vi "Vision Processing.vi"(4 "error in (no error)":errorcluster, 7 "Image Size":T1=enum."320x240") -> ()   [LabVIEW 2013]
doc: "This VI runs in parallel to other tasks. It gets images from the camera, processes them for color or shape and use that information to affect robot behavior."
uses:
  <vilib>/Rock Robotics/WPI/Camera/WPI_CameraImageSize.ctl
  <vilib>/Rock Robotics/WPI/Camera/WPI_CameraWhite Balance Values.ctl
  <vilib>/Rock Robotics/WPI/Camera/WPI_CameraExposure Values.ctl
  <vilib>/Rock Robotics/WPI/Camera/WPI_CameraFrameRate.ctl
  Robot Global Data.vi
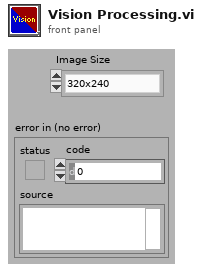
[diagram p1: front panel]
types:
  T1 = typedef "WPI_CameraImageSize.ctl" = enum16{"640x480", "320x240", "160x120"}
  T2 = typedef "WPI_CameraFrameRate.ctl" = u32
  T3 = typedef "WPI_CameraExposure Values.ctl" = enum16{"Auto", "Flicker-free 50 Hz", "Flicker-free 60 Hz", "Hold current"}
  T4 = typedef "WPI_CameraWhite Balance Values.ctl" = enum16{"Auto", "Fixed indoor", "Fixed outdoor 1", "Fixed outdoor 2", "Fixed fluorescent 1", "Fixed fluorescent 2", "Hold current"}
  T5 = typedef "Image Type" = u32
  T6 = typedef "WPI_CameraDevRef.ctl" = cluster{"Camera Address":string, "CameraStatus":errorcluster, "Acquire Image Notifier":refnum<notifier>}
  T7 = typedef "IMAQ Image.ctl" = refnum<image>
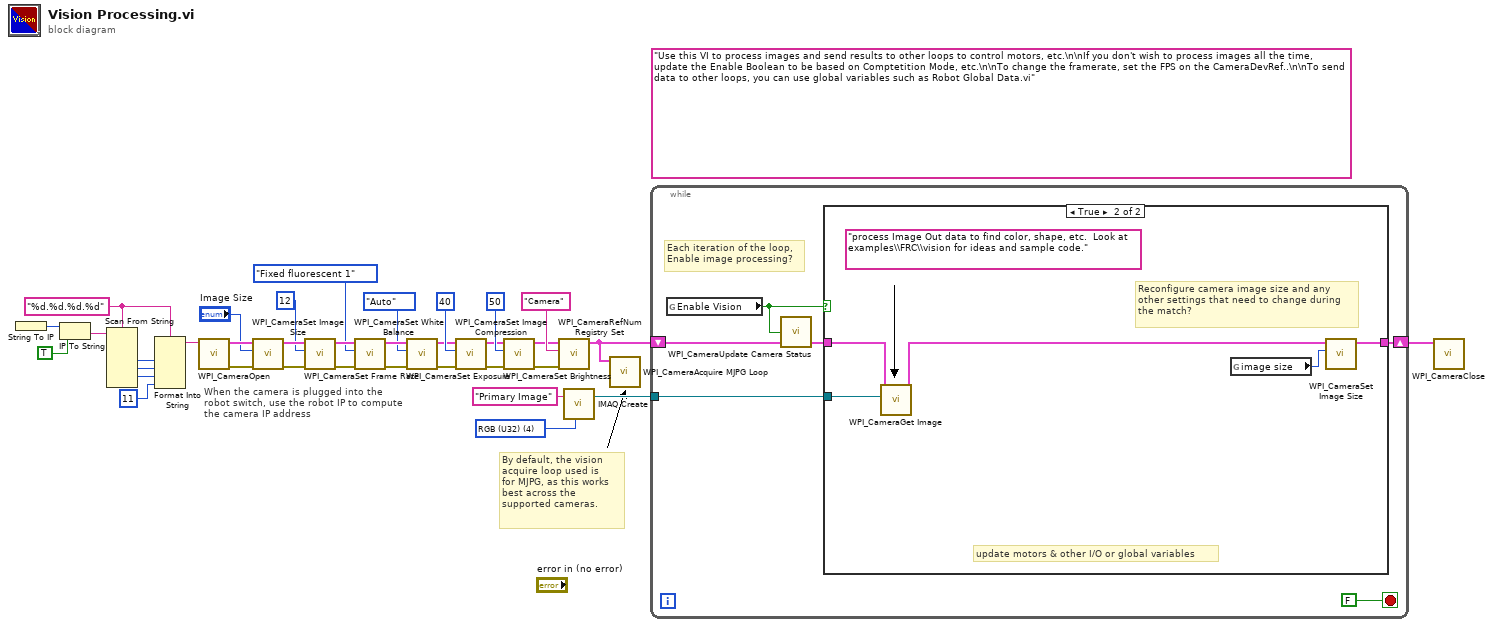
[diagram p0: block diagram]
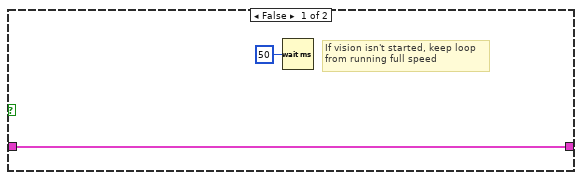
[diagram p2: hidden frame]
diagram:
  w5 = "%d.%d.%d.%d" ("format string")
  (unwired) "Use this VI to process images and send results to other loops to control motors, etc.\n\nIf you don't wish to process images all the time, update the Enable Boolean to be based on Comptetition Mode, etc.\n\nTo change the framerate, set the FPS on the CameraDevRef..\n\nTo send data to other loops, you can use global variables such as Robot Global Data.vi"
  w35 = T5 4 items=["Grayscale (U8)", "Grayscale (I16)", "Grayscale (SGL)", "Complex (CSG)", "RGB (U32)", "HSL (U32)", "RGB (U64)"] ("Image Type")
  # "When the camera is plugged into the\nrobot switch, use the robot IP to compute\nthe camera IP address"
  # "By default, the vision\nacquire loop used is\nfor MJPG, as this works\nbest across the\nsupported cameras."
  n1 = String To IP() -> (0:w12:u32)  [unwired: 1 in]
  n2 = IP To String(1:TRUE ("dot notation? (F)"), 2:w12) -> (0:w10:string)
  n3 = Scan From String(format string=w5, input string=w10) -> (output 1=w9:i32, output 2=w8:i32, output 3=w7:i32)  [unwired: 7 in, 3 out]
  n4 = Format Into String(format string=w5, w9, w8, w7, 11 ("Compression")) -> (resulting string=w4:string)  [unwired: 2 in, 1 out]
  n5 = call <vilib>:"WPI_CameraOpen.vi"("Camera Address"=w4) -> ("error out"=w23:errorcluster, "CameraDevRef"=w24:T6)  [unwired: 1 in, 8 out]
  n6 = call <vilib>:"WPI_CameraSet Image Size.vi"("error in (no error)"=w23, "Image Size"="Image Size", "CameraDevRef"=w24) -> ("error out"=w22:errorcluster, "CameraDevRef Out"=w25:T6)  [unwired: 7 out]
  n7 = call <vilib>:"WPI_CameraSet Frame Rate.vi"("error in (no error)"=w22, "Frame Rate (fps)"=T2 12, "CameraDevRef"=w25) -> ("error out"=w21:errorcluster, "CameraDevRef Out"=w27:T6)  [unwired: 7 out]
  n8 = call <vilib>:"WPI_CameraSet White Balance.vi"("error in (no error)"=w21, "White Balance"=WPI_CameraWhite_Balance_Values."Fixed fluorescent 1", "CameraDevRef"=w27) -> ("error out"=w20:errorcluster, "CameraDevRef Out"=w26:T6)  [unwired: 7 out]
  n9 = call <vilib>:"WPI_CameraSet Exposure.vi"("error in (no error)"=w20, "Exposure"=WPI_CameraExposure_Values."Auto", "CameraDevRef"=w26) -> ("error out"=w19:errorcluster, "CameraDevRef Out"=w29:T6)  [unwired: 7 out]
  n10 = call <vilib>:"WPI_CameraSet Image Compression.vi"("error in (no error)"=w19, "Compression"=40, "CameraDevRef"=w29) -> ("error out"=w18:errorcluster, "CameraDevRef Out"=w28:T6)  [unwired: 7 out]
  n11 = call <vilib>:"WPI_CameraSet Brightness.vi"("error in (no error)"=w18, "Brightness"=50, "CameraDevRef"=w28) -> ("error out"=w16:errorcluster, "CameraDevRef Out"=w17:T6)  [unwired: 7 out]
  n12 = call <vilib>:"WPI_CameraRefNum Registry Set.vi"("error in (no error)"=w16, "refnum name"="Camera", "CameraDevRef"=w17) -> ("CameraDevRef"=w3:T6)  [unwired: 8 out]
  n13 = call "IMAQ Create"("Image Name"="Primary Image", "Image Type"=w35) -> ("New Image"=w33:T7)  [unwired: 2 in, 2 out]
  n14 = call <vilib>:"WPI_CameraAcquire MJPG Loop.vi"("CameraDevRef"=w3) -> ()  [unwired: 11 in]
  n15 = while {
    shift-right: [w40] -> w1
    shift-left: w3 -> [w38]
    tunnel: w33 -> [w39]
    stop <- FALSE stop-if-true
    # "Each iteration of the loop,\nEnable image processing?"
    n16 = global read "Robot Global Data.vi" "Enable Vision"() -> (w36:bool)
    n17 = call <vilib>:"WPI_CameraUpdate Camera Status.vi"("CameraDevRef In"=w38, "Enable Vision"=w36) -> ("CameraDevRef Out"=w37:T6)  [unwired: 3 in]
    n18 = case shown="True" w36 {
      tunnel: w39 -> [_ w47]
      tunnel: [w43 w48] -> w40
      tunnel: w37 -> [w43 w45]
      frame False {
        # "If vision isn't started, keep loop\nfrom running full speed"
        n19 = Wait (ms)(milliseconds to wait=u32 50) -> ()  [unwired: 1 out]
      }
      frame True {
        (unwired) "process Image Out data to find color, shape, etc.  Look at examples\\FRC\\vision for ideas and sample code."
        # "update motors & other I/O or global variables"
        # "Reconfigure camera image size and any\nother settings that need to change during\nthe match?"
        n20 = call <vilib>:"WPI_CameraGet Image.vi"("Image"=w47, "CameraDevRef"=w45) -> ("CameraDevRef Out"=w44:T6)  [unwired: 1 in, 8 out]
        n21 = global read "Robot Global Data.vi" "image size"() -> (w46:T1)
        n22 = call <vilib>:"WPI_CameraSet Image Size.vi"("Image Size"=w46, "CameraDevRef"=w44) -> ("CameraDevRef Out"=w48:T6)  [unwired: 1 in, 8 out]
      }
    }
  }
  n23 = call <vilib>:"WPI_CameraClose.vi"("CameraDevRef"=w1) -> ()  [unwired: 1 in, 10 out]
